vi "Parse FPGA Bitfile.vi"(8 "error in (no error)":errorcluster, 11 "Path":path) -> (0 "error out":errorcluster, 2 "DMA configuration array":T8[](array[typedef])=[{"Name"="P2PSource", "Depth"=1023, "Write? (Deprecated:Use Implementation)"=TRUE, "Physical Channel"=0, "Base Address"=65472, "Data Width"=32, "Data Type"=enum."U32", "FXP Properties"=variant(fxp<+,32,32> 0.0), "Write Window Address"=0, "Implementation"=enum."niFpgaPeerToPeerWriter", "Control Set"=0}, {"Name"="P2PSink", "Depth"=1023, "Write? (Deprecated:Use Implementation)"=FALSE, "Physical Channel"=1, "Base Address"=65408, "Data Width"=32, "Data Type"=enum."U32", "FXP Properties"=variant(fxp<+,32,32> 0.0), "Write Window Address"=57344, "Implementation"=enum."niFpgaPeerToPeerReader", "Control Set"=1}], 3 "vi info":T1 {"RegisterMap"."Address" format="%.0x"})   [LabVIEW 2019, in "FPGA Addon System Explorer.lvlib"]
uses:
  FPGA Addon System Explorer.lvlib
  <vilib>/rvi/FIFO/Fifo_Types/Fifo_DMA_Config.ctl
  <vilib>/rvi/DataTransferAndStorage/Container/Common/niFpgaDataTypeControl.ctl
  <vilib>/rvi/ClientSDK/Core/ModuleGeneration/CommunicationInterfaceUtility/niFpgaDmaChannelImplementation.ctl
  <vilib>/rvi/Bitfile/niFpgaBitfileStructure_VI.ctl
  <vilib>/rvi/Bitfile/nirviControlStructure.ctl
  <vilib>/rvi/Bitfile/nirviTypdefDescription.ctl
  <vilib>/rvi/Bitfile/nirviMechanicalAction.ctl
  <vilib>/rvi/Bitfile/nirviSubControlStructure.ctl
  <vilib>/rvi/Bitfile/nirviClusterElementControl.ctl
  <vilib>/picture/picture.llb/imagedata.ctl
  <vilib>/rvi/ClientSDK/Host Interface/DMA/public/niFpgaDmaChannelVisibilityFilter.ctl
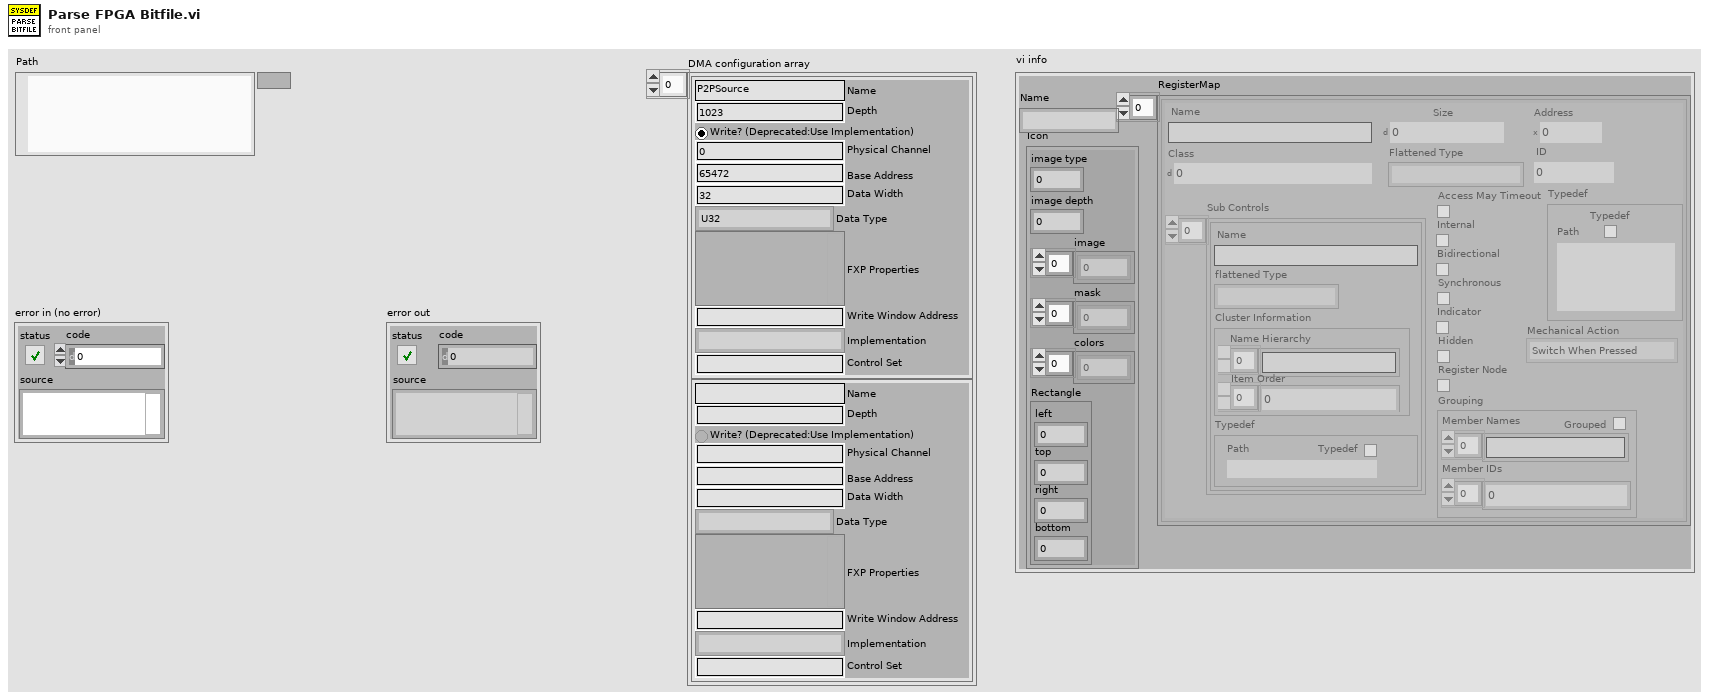
[diagram p1: front panel]
types:
  T1 = typedef "niFpgaBitfileStructure_VI.ctl" = cluster{"Name":string, "RegisterMap":T2[], "Icon":T7}
  T2 = typedef "nirviControlStructure.ctl" = cluster{"Name":string, "Hidden":bool, "Indicator":bool, "Flattened Type":string, "Grouping":cluster{"Grouped":bool, "Member Names":string[], "Member IDs":u32[]}, "Address":u32, "Size":u32, "Class":u32, "Internal":bool, "Typedef":T3, "ID":u32, "Bidirectional":bool, "Synchronous":bool, "Mechanical Action":T4, "Sub Controls":T5[], "Access May Timeout":bool, "Register Node":bool}
  T3 = typedef "nirviTypdefDescription.ctl" = cluster{"Typedef":bool, "Path":path}
  T4 = typedef "nirviMechanicalAction.ctl" = enum8{"Switch When Pressed", "Switch When Released", "Switch Until Released", "Latch When Pressed", "Latch When Released", "Latch Until Released"}
  T5 = typedef "nirviSubControlStructure.ctl" = cluster{"Name":string, "flattened Type":string, "Cluster Information":T6, "Typedef":T3}
  T6 = typedef "nirviClusterElementControl.ctl" = cluster{"Name Hierarchy":string[], "Item Order":u32[]}
  T7 = typedef "imagedata.ctl" = cluster{"image type":i32, "image depth":i32, "image":u8[], "mask":u8[], "colors":u32[], "Rectangle":cluster{"left":i16, "top":i16, "right":i16, "bottom":i16}}
  T8 = typedef "Fifo_DMA_Config.ctl" = cluster{"Name":string, "Depth":u32, "Write? (Deprecated:Use Implementation)":bool, "Physical Channel":u32, "Base Address":u32, "Data Width":u32, "Data Type":T9, "FXP Properties":variant, "Write Window Address":u32, "Implementation":T10, "Control Set":u32}
  T9 = typedef "niFpgaDataTypeControl.ctl" = enum32{"Boolean", "I8", "I16", "I32", "I64", "U8", "U16", "U32", "U64", "FXP", "CustomControl", "SGL"}
  T10 = typedef "niFpgaDmaChannelImplementation.ctl" = enum16{"niFpgaTargetToHost", "niFpgaHostToTarget", "niFpgaPeerToPeerWriter", "niFpgaPeerToPeerReader", "niCoreTargetToHost", "niCoreHostToTarget"}
  T11 = typedef "niFpgaDmaChannelVisibilityFilter.ctl" = enum16{"All", "UserVisible"}
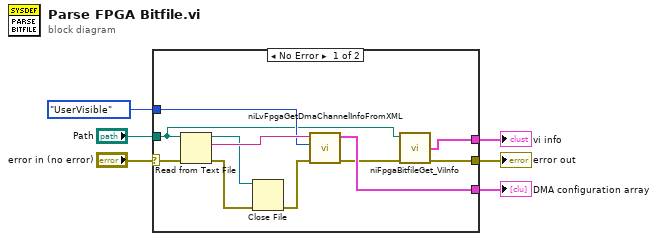
[diagram p0: block diagram]
diagram:
  n1 = case shown="No Error" "error in (no error)" {
    selector: "error in (no error)" -> [w13 w18]
    tunnel: [w8 w18] -> w5
    tunnel: "Path" -> [w10 _]
    tunnel: niFpgaDmaChannelVisibilityFilter."UserVisible" ("DMA Channel Filter") -> [w12 _]
    tunnel: [w7 _] -> w1
    tunnel: [w11 _] -> w2
    frame No Error {
      n2 = Read from Text File(file (use dialog)=w10, error in=w13) -> (refnum out=w16:refnum<file>, text=w17:string, error out=w15:errorcluster)  [unwired: 3 out]
      n3 = Close File(refnum=w16, error in=w15) -> (error out=w14:errorcluster)  [unwired: 1 out]
      n4 = call <resource>:"niLvFpgaGetDmaChannelInfoFromXML.vi"("error in (no error)"=w14, "DMA Channel Filter"=w12, "XML String in"=w17) -> ("error out"=w9:errorcluster, "DMA configuration array"=w11:T8[])  [unwired: 7 out]
      n5 = call <vilib>:"niFpgaBitfileGet_ViInfo.vi"("bitfile path"=w10, "error in (no error)"=w9) -> ("vi info"=w7:T1, "error out"=w8:errorcluster)  [unwired: 1 in, 11 out]
    }
    frame Error {
    }
  }
  "error out" <- w5
  "DMA configuration array" <- w2
  "vi info" <- w1
